vi "Get Color (Hex).vi"(8 "error in (no error)":errorcluster, 11 "Style in":refnum<class "Style.lvclass">) -> (0 "error out":errorcluster, 2 "Color (Hex)":string, 3 "Style out":refnum<class "Style.lvclass">)   [LabVIEW 2017, in "Styles.lvlib" / "Style.lvclass"]
uses:
  Style.lvclass
  Style.lvclass/Style.ctl
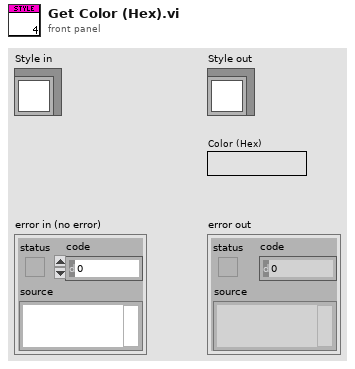
[diagram p1: front panel]
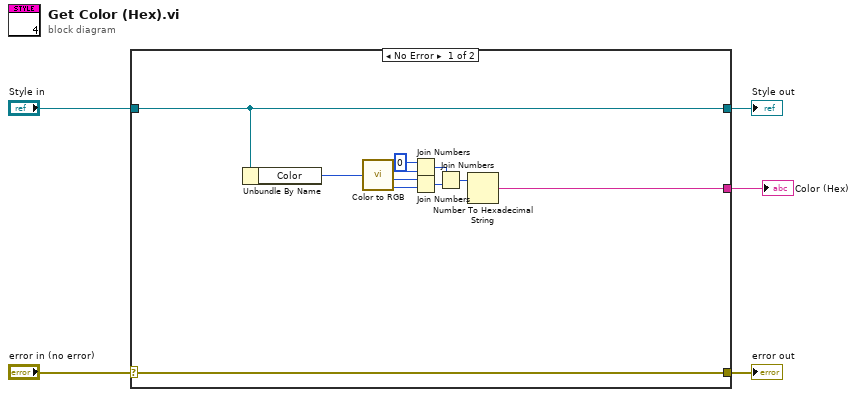
[diagram p0: block diagram]
diagram:
  n1 = case shown="No Error" "error in (no error)" {
    selector: "error in (no error)" -> [w16 w18]
    tunnel: [w16 w18] -> w4
    tunnel: [w15 w17] -> w2
    tunnel: "Style in" -> [w15 w17]
    tunnel: [w6 _] -> w1
    frame No Error {
      n2 = Unbundle By Name(w15) -> ("Color"=w7:u32)
      n3 = call <vilib>:"Color to RGB.vi"("Color"=w7) -> ("R"=w14:u8, "G"=w13:u8, "B"=w12:u8)  [unwired: 1 out]
      n4 = Join Numbers(hi=u8 0, lo=w14) -> ((hi.lo)=w10:u16)
      n5 = Join Numbers(hi=w13, lo=w12) -> ((hi.lo)=w9:u16)
      n6 = Join Numbers(hi=w10, lo=w9) -> ((hi.lo)=w8:u32)
      n7 = Number To Hexadecimal String(2:w8) -> (0:w6:string)  [unwired: 1 in]
    }
    frame Error {
    }
  }
  "error out" <- w4
  "Style out" <- w2
  "Color (Hex)" <- w1
